vi "main.vi"() -> ()   [LabVIEW 2016]
panel:
  out "Tank Full":bool
  out "Valve":bool
  out "Slide":u8(slide) scale=0.0..10.0
  out "Tank 2":dbl(slide) scale=0.0..10.0
  out "Tank":dbl(slide) scale=0.0..10.0
  out "Slide 2":u8(slide)
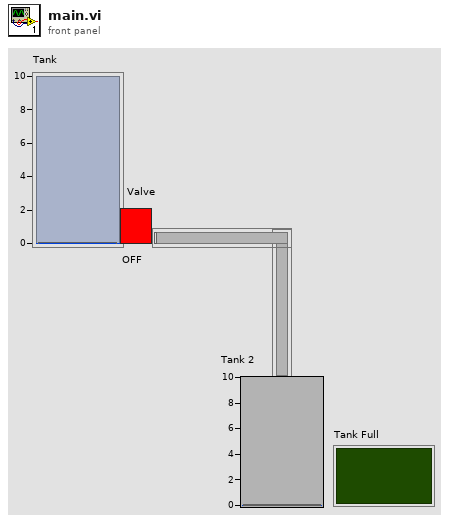
[diagram p1: front panel]
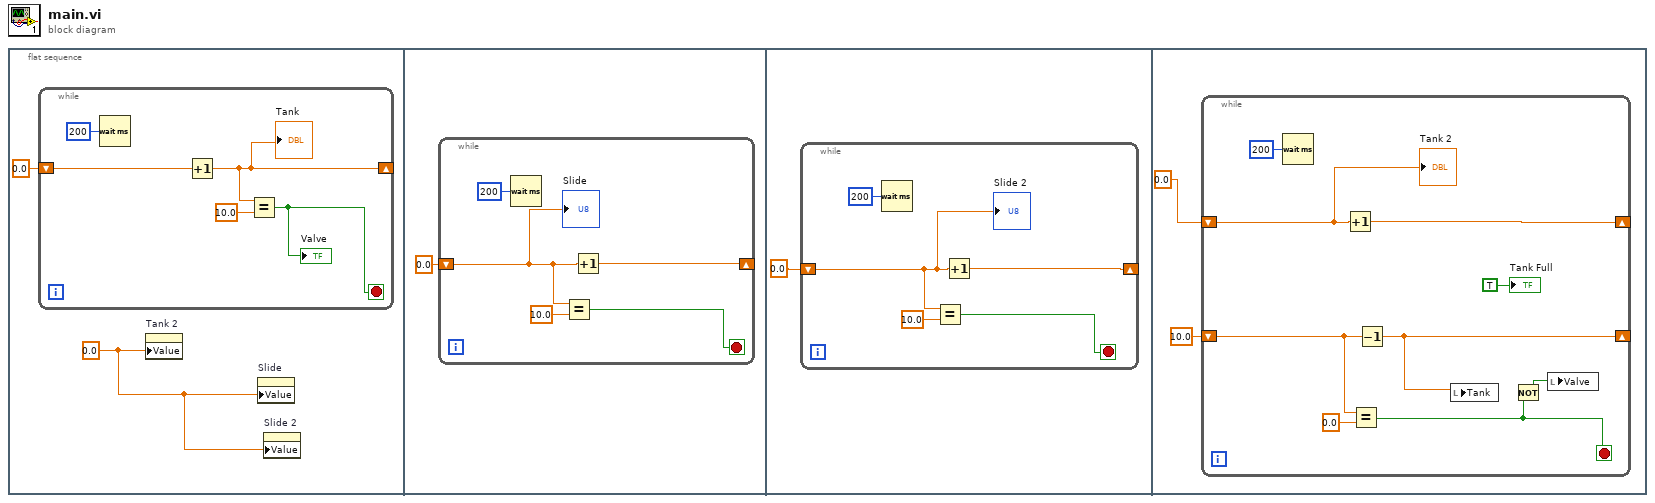
[diagram p0: block diagram]
diagram:
  n1 = flat-sequence {
    frame #0 {
      w1 = 0.0 ("Tank 2")
      n2 = while {
        shift-right: [w6] -> _
        shift-left: 0.0 -> [w7]
        stop <- w3 stop-if-true
        n3 = Wait (ms)(milliseconds to wait=u32 200) -> ()  [unwired: 1 out]
        n4 = Increment(x=w7) -> (x+1=w6:dbl)
        "Tank" <- w6
        n5 = Equal?(x=w6, y=10.0) -> (x = y?=w3:bool)
        "Valve" <- w3
      }
      n6 = property on="Tank 2" class="Slide (strict)"("Value"=w1) -> ()  [unwired: 2 in, 2 out]
      n7 = property on="Slide" class="Slide (strict)"("Value"=w1) -> ()  [unwired: 2 in, 2 out]
      n8 = property on="Slide 2" class="Slide (strict)"("Value"=w1) -> ()  [unwired: 2 in, 2 out]
    }
    frame #1 {
      n9 = while {
        shift-right: [w13] -> _
        shift-left: 0.0 -> [w12]
        stop <- w10 stop-if-true
        n10 = Wait (ms)(milliseconds to wait=u32 200) -> ()  [unwired: 1 out]
        n11 = Equal?(x=w12, y=10.0) -> (x = y?=w10:bool)
        n12 = Increment(x=w12) -> (x+1=w13:dbl)
        "Slide" <- w12
      }
    }
    frame #2 {
      n13 = while {
        shift-right: [w19] -> _
        shift-left: 0.0 -> [w15]
        stop <- w17 stop-if-true
        n14 = Wait (ms)(milliseconds to wait=u32 200) -> ()  [unwired: 1 out]
        n15 = Equal?(x=w15, y=10.0) -> (x = y?=w17:bool)
        n16 = Increment(x=w15) -> (x+1=w19:dbl)
        "Slide 2" <- w15
      }
    }
    frame #3 {
      n17 = while {
        shift-right: [w30] -> _
        shift-left: 0.0 -> [w28]
        shift-right: [w27] -> _
        shift-left: 10.0 -> [w25]
        stop <- w23 stop-if-true
        n18 = Wait (ms)(milliseconds to wait=u32 200) -> ()  [unwired: 1 out]
        n19 = Increment(x=w28) -> (x+1=w30:dbl)
        n20 = Equal?(x=w25, y=0.0) -> (x = y?=w23:bool)
        n21 = Decrement(x=w25) -> (x-1=w27:dbl)
        n22 = local write "Tank"(w27) -> ()
        n23 = Not(x=w23) -> (.not. x?=w22:bool)
        n24 = local write "Valve"(w22) -> ()
        "Tank 2" <- w28
        "Tank Full" <- TRUE ("Tank Full")
      }
    }
  }
